vi "LibraryLogging.vi"(7 "LJM_DEBUG_LOG_BUFFER_MAX_SIZE":i32, 8 "error in":errorcluster, 9 "LJM_DEBUG_LOG_LEVEL":i32, 10 "LJM_DEBUG_LOG_MODE":i32) -> (0 "error out":errorcluster)   [LabVIEW 2024]
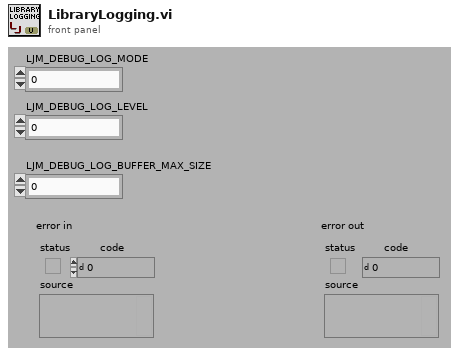
[diagram p1: front panel]
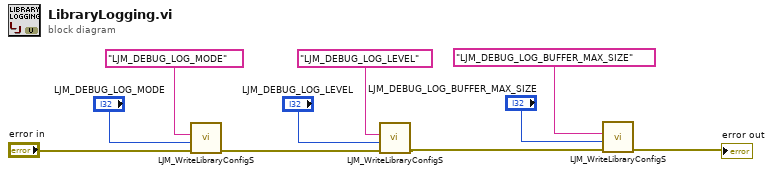
[diagram p0: block diagram]
diagram:
  n1 = call "LJM_WriteLibraryConfigS.vi"("error in"="error in", "Value"="LJM_DEBUG_LOG_MODE", "Parameter"="LJM_DEBUG_LOG_MODE") -> ("error out"=w5:errorcluster)  [unwired: 8 in]
  n2 = call "LJM_WriteLibraryConfigS.vi"("error in"=w5, "Value"="LJM_DEBUG_LOG_LEVEL", "Parameter"="LJM_DEBUG_LOG_LEVEL") -> ("error out"=w2:errorcluster)  [unwired: 8 in]
  n3 = call "LJM_WriteLibraryConfigS.vi"("error in"=w2, "Value"="LJM_DEBUG_LOG_BUFFER_MAX_SIZE", "Parameter"="LJM_DEBUG_LOG_BUFFER_MAX_SIZE") -> ("error out"=→"error out":errorcluster)  [unwired: 8 in]
